vi "Export Experiment Data.vi"(6 "V to AU Conversion":dbl, 8 "Samples Per Average":i32, 9 "Skip Export":bool, 10 "Export?":bool, 11 "Data":dbl[][](array[numeric])) -> (3 "Export Complete?":bool)   [LabVIEW 2016]
uses:
  <vilib>/Utility/error.llb/DialogType.ctl
  <vilib>/Utility/file.llb/Write Delimited Spreadsheet (string).vi
  <vilib>/Utility/file.llb/Write Delimited Spreadsheet (DBL).vi
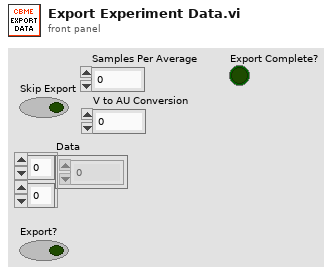
[diagram p1: front panel]
types:
  T1 = enum16{"open", "replace", "create", "open or create", "replace or create", "replace or create with confirmation"}
  T2 = typedef "DialogType.ctl" = u16
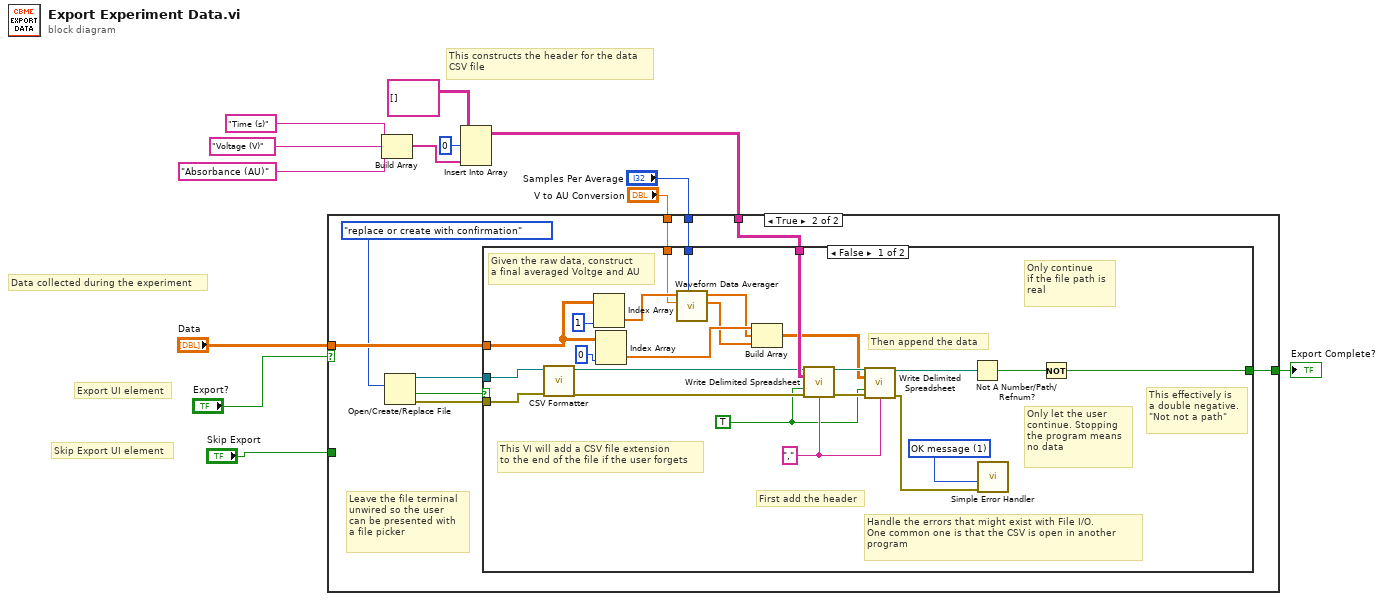
[diagram p0: block diagram]
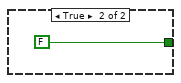
[diagram p3: hidden frame]
diagram:
  # "Skip Export UI element"
  # "Export UI element"
  # "Data collected during the experiment"
  # "This constructs the header for the data\nCSV file"
  n1 = Build Array("Time (s)", "Voltage (V)", "Absorbance (AU)") -> (w8:string[])
  n2 = Insert Into Array(array=string[][] [], index (row)=0, new element=w8) -> (w11:string[][])  [unwired: 1 in]
  n3 = case shown="True" "Export?" {
    tunnel: "Data" -> [_ w22]
    tunnel: [w14 w23] -> w3
    tunnel: "Skip Export" -> [w14 _]
    tunnel: w11 -> [_ w21]
    tunnel: "Samples Per Average" -> [_ w16]
    tunnel: "V to AU Conversion" -> [_ w15]
    frame False {
      # "The user doesn't want to export,\nso skip this step"
    }
    frame True {
      # "Leave the file terminal \nunwired so the user \ncan be presented with \na file picker"
      n4 = Open/Create/Replace File(operation (0:open)=T1."replace or create with confirmation") -> (refnum out=w17:refnum<file>, cancelled=w19:bool, error out=w18:errorcluster)  [unwired: 5 in]
      n5 = case shown="False" w19 {
        tunnel: [w45 FALSE] -> w23
        tunnel: w22 -> [w31 _]
        tunnel: w21 -> [w42 _]
        tunnel: w18 -> [w38 _]
        tunnel: w17 -> [w37 _]
        tunnel: w16 -> [w25 _]
        tunnel: w15 -> [w24 _]
        frame False {
          w39 = T2 1 items=["no dialog", "OK message", "continue or stop message", "OK message + warnings", "continue/stop + warnings"] ("type of dialog (OK msg:1)")
          w35 = TRUE ("append to file? (new file:F)")
          w41 = "," ("delimiter (\\t)")
          # "Given the raw data, construct\na final averaged Voltge and AU"
          # "This VI will add a CSV file extension\nto the end of the file if the user forgets"
          # "Only let the user\ncontinue. Stopping\nthe program means\nno data"
          # "Handle the errors that might exist with File I/O.\nOne common one is that the CSV is open in another\nprogram"
          # "This effectively is\na double negative.\n\"Not not a path\""
          # "Only continue\nif the file path is \nreal"
          # "Then append the data"
          # "First add the header"
          n6 = call "CSV Formatter.vi"("error in (no error)"=w38, "Byte Stream File in"=w37) -> ("error out"=w36:errorcluster, "path"=w34:path)  [unwired: 8 in]
          n7 = Index Array(array=w31, index (col)=1 ("disabled index (col)")) -> (element=w32:dbl[])  [unwired: 1 in]
          n8 = Index Array(array=w31, index (col)=0 ("disabled index (col)")) -> (element=w29:dbl[])  [unwired: 1 in]
          n9 = call "Waveform Data Averager.vi"("Samples Per Average"=w25, "V to AU Conversion"=w24, "Voltage Array In"=w32) -> ("AU Array Out"=w27:dbl[], "Voltage Array Out"=w28:dbl[])  [unwired: 7 in]
          n10 = Build Array(w29, w28, w27) -> (w26:dbl[][])
          n11 = call-poly <vilib>:"Write Delimited Spreadsheet.vi"("file path (dialog if empty)"=w34, "2D data"=w42, "append to file? (new file:F)"=w35, "error in (no error)"=w36, "delimiter (\\t)"=w41) -> ("new file path (Not A Path if cancelled)"=w44:path, "error out"=w43:errorcluster)  [unwired: 9 in]
          n12 = call-poly <vilib>:"Write Delimited Spreadsheet.vi"("file path (dialog if empty)"=w44, "2D data"=w26, "append to file? (new file:F)"=w35, "error in (no error)"=w43, "delimiter (\\t)"=w41) -> ("new file path (Not A Path if cancelled)"=w47:path, "error out"=w40:errorcluster)  [unwired: 9 in]
          n13 = Not A Number/Path/Refnum?(number/path/refnum=w47) -> (NaN/Path/Refnum?=w46:bool)
          n14 = call <vilib>:"Simple Error Handler.vi"("type of dialog (OK msg:1)"=w39, "error in (no error)"=w40) -> ()  [unwired: 3 in, 5 out]
          n15 = Not(x=w46) -> (.not. x?=w45:bool)
        }
        frame True {
        }
      }
    }
  }
  "Export Complete?" <- w3
